vi "Delay.vi"(8 "No Error":errorcluster, 11 "ms":u32) -> (0 "error out":errorcluster)   [LabVIEW 2026, in "SDL3.lvlib" / "Timer.lvlib"]
doc: "<B>Summary</B>\nWait a specified number of milliseconds before returning.\n\n<B>Remarks</B>\nThis function waits a specified number of milliseconds before returning. It waits at least the specified time, but possibly longer due to OS scheduling."
uses:
  Timer.lvlib
  Lib/SDL3.dll
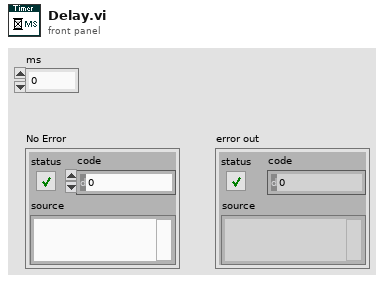
[diagram p1: front panel]
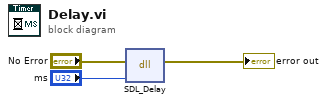
[diagram p0: block diagram]
diagram:
  n1 = dll-call lib="C:/Users/saukko/Dev/LV-SDL3/Sources/SDL3/Lib/SDL3.*" fn="SDL_Delay"(error in="No Error", "ms"="ms") -> (error out=→"error out":errorcluster)  [unwired: 4 in, 1 out]
